vi "Read Command Status.vi"(8 "error in (no error)":errorcluster, 11 "Command in":refnum<class "Command State Actor.lvclass">) -> (0 "error out":errorcluster, 2 "Command Status":T1, 3 "Command out":refnum<class "Command State Actor.lvclass">)   [LabVIEW 2013, in "Command State Actor.lvlib" / "Command State Actor.lvclass"]
uses:
  Command State Actor.lvclass
  Command Status.ctl
  Command States.ctl
  State Status.ctl
  Command State Actor.lvclass/Command State Actor.ctl
  Command Actor/Command States/Command States.lvclass
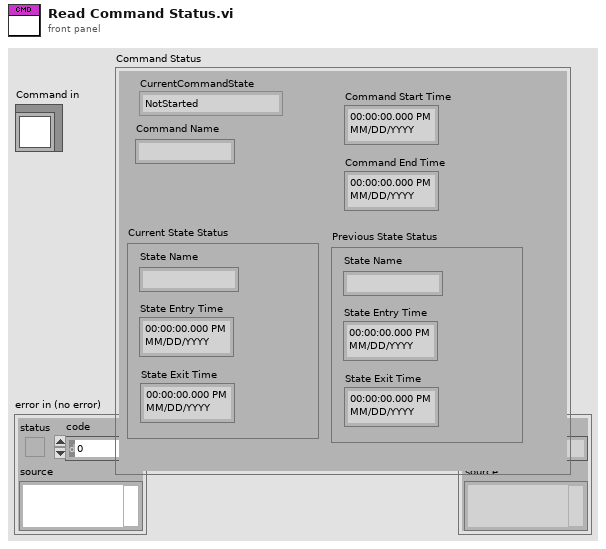
[diagram p1: front panel]
types:
  T1 = typedef "Command State Actor.lvlib/Command State Actor.lvclass/Command Status.ctl" = cluster{"CurrentCommandState":T2, "Command Name":string, "Current State Status":T3, "Command Start Time":timestamp, "Command End Time":timestamp, "Previous State Status":T3}
  T2 = typedef "Command State Actor.lvlib/Command State Actor.lvclass/Command States.ctl" = enum16{"NotStarted", "Starting", "Started", "Executing", "Completing", "Completed", "Stopping", "Stopped"}
  T3 = typedef "Command Actor.lvlib/Command States.lvclass/State Status.ctl" = cluster{"State Name":string, "State Entry Time":timestamp, "State Exit Time":timestamp}
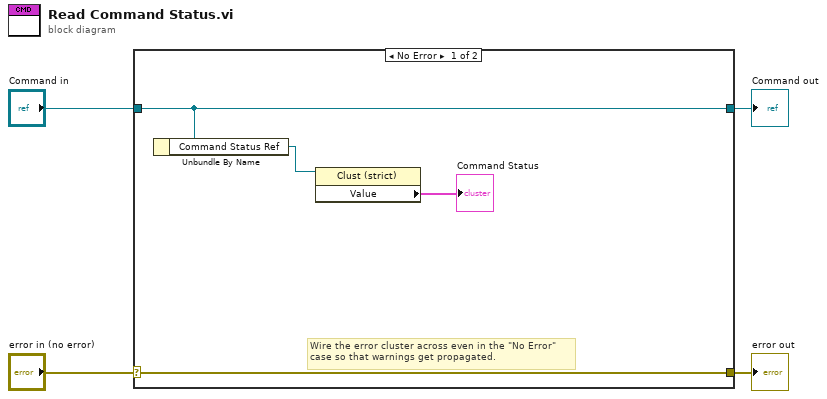
[diagram p0: block diagram]
diagram:
  n1 = case shown="No Error" "error in (no error)" {
    selector: "error in (no error)" -> [w8 w10]
    tunnel: [w8 w10] -> w3
    tunnel: [w7 w9] -> w1
    tunnel: "Command in" -> [w7 w9]
    frame No Error {
      # "Wire the error cluster across even in the \"No Error\"\ncase so that warnings get propagated."
      n2 = Unbundle By Name(w7) -> ("Command Status Ref"=w6:refnum<vi>)
      n3 = property class="Clust (strict)"(reference=w6) -> ("Value"=→"Command Status":T1)  [unwired: 1 in, 2 out]
    }
    frame Error {
    }
  }
  "error out" <- w3
  "Command out" <- w1
